vi "CSGaussmeter.saveSetting.vi"(0 "i ref in":refnum<vi>, 7 "ms timeout (10000)":i32=10000, 9 "setting path":string, 11 "error in (no error)":errorcluster) -> (4 "i ref out":refnum<vi>, 8 "timed out":bool, 15 "error out":errorcluster)   [LabVIEW 2014, in "CSGaussmeter.lvlib"]
uses:
  CSGaussmeter.lvlib
  CS_Core/CSObj/CSObj.lvlib
  CSlibraries/UtilityLib/UtilityLib.lvlib
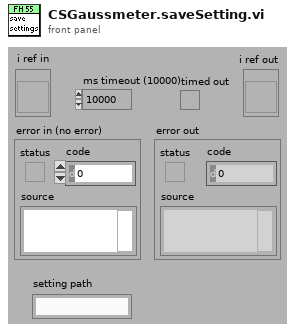
[diagram p1: front panel]
types:
  T1 = enum16{"open", "replace", "create", "open or create", "replace or create", "replace or create with confirmation"}
  T2 = typedef "CSGaussmeter.lvlib/CSGaussmeter.i attribute.ctl" = cluster{"Name":string, "VISA Resource Name":refnum<visa-resource-name>, "actValues":cluster{" Limit":bool, "Unit ":T3, "Temp_Unit":T4, "Max":T5, " Filter":bool, " Peak":bool, " Auto_Range":bool, "Range":T6, " Rel":bool, " CTemp":bool, " CField":bool, "AC_DC ":bool, "Set_lower":cluster{"Numeric":dbl, "Cancel Button":bool, "Unit":T7}, "Set_upper":cluster{"Numeric":dbl, "Cancel Button":bool, "Unit":T7}, "Set_Rel":cluster{"Numeric":dbl, "Cancel Button":bool, "Unit":T7}, "Zero":bool, " Local":bool, "Reset":bool, " Init":bool}, "FH 55 Gauss-/Teslameter":T8, "MAX_Value":T9, "MIN_Value":T9, "Rel_Value":T9, "Array ":string[], "LIMU":dbl, " LIML":dbl, "Messwerte 2":string, "Messwerte ":cluster{"Numeric":i32, "OK Button":bool}, "serviceID":cluster{"Current ID":i32, "Unit ID":i32, "Temp ID":i32, "Name ID \n":i32, "Visa ID ":i32}, "setValues ":cluster{" Limit":bool, "Unit ":T3, "Temp_Unit":T4, "Max":T5, " Filter":bool, " Peak":bool, " Auto_Range":bool, "Range":T6, " Rel":bool, " CTemp":bool, " CField":bool, "AC_DC ":bool, "Set_lower":cluster{"Numeric":dbl, "Cancel Button":bool, "Unit":T7}, "Set_upper":cluster{"Numeric":dbl, "Cancel Button":bool, "Unit":T7}, "Set_Rel":cluster{"Numeric":dbl, "Cancel Button":bool, "Unit":T7}, "Zero":bool, " Local":bool, "Reset":bool, " Init":bool}}
  T3 = typedef "FH 55.lvlib/Unit.ctl" = enum16{"T", "G", "A/m"}
  T4 = typedef "FH 55.lvlib/Temp_Unit.ctl" = enum16{"Temp off", "Celsius", "Fahrenheit"}
  T5 = typedef "FH 55.lvlib/Max.ctl" = enum16{"MAX off", "Show MAX", "MAX/MIN"}
  T6 = typedef "FH 55.lvlib/Range.ctl" = enum16{"1", "2", "3", "4", "5", "6", "7"}
  T7 = typedef "FH 55.lvlib/Unit2.ctl" = enum16{"mT", "G", "kA/m"}
  T8 = typedef "FH 55.lvlib/Display.ctl" = cluster{"current value":string, "Limit":string, "Remote":string, "function ":string, "Cluster":cluster{"AC/DC":string, "Auto":string, "Filter":string, "Range":string, "Rel":string, "Peak":string}}
  T9 = typedef "FH 55.lvlib/Value_String.ctl" = cluster{"Numeric":dbl, "String":string}
  T10 = cluster{" Limit":bool, "Unit ":T3, "Temp_Unit":T4, "Max":T5, " Filter":bool, " Peak":bool, " Auto_Range":bool, "Range":T6, " Rel":bool, " CTemp":bool, " CField":bool, "AC_DC ":bool, "Set_lower":cluster{"Numeric":dbl, "Cancel Button":bool, "Unit":T7}, "Set_upper":cluster{"Numeric":dbl, "Cancel Button":bool, "Unit":T7}, "Set_Rel":cluster{"Numeric":dbl, "Cancel Button":bool, "Unit":T7}, "Zero":bool, " Local":bool, "Reset":bool, " Init":bool}
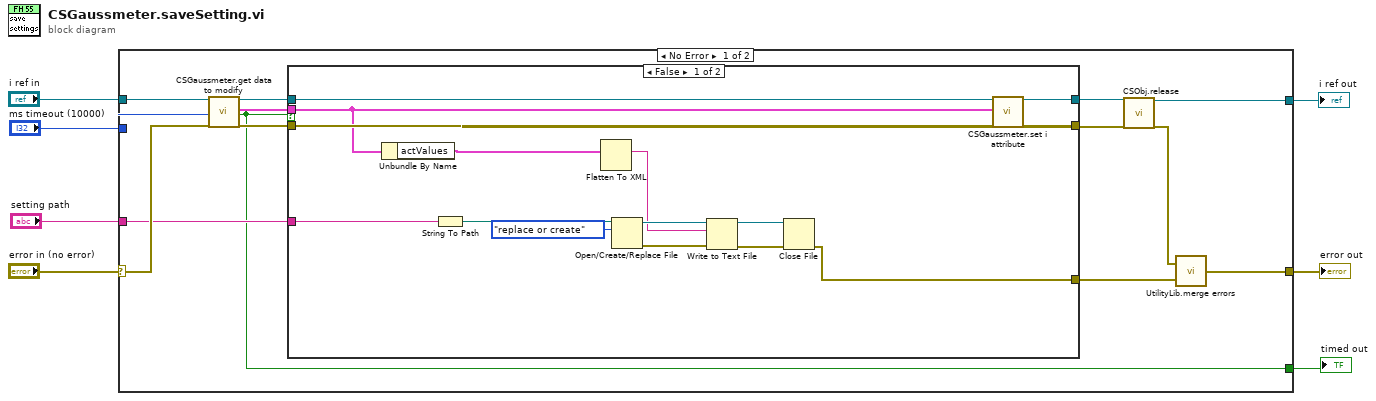
[diagram p0: block diagram]
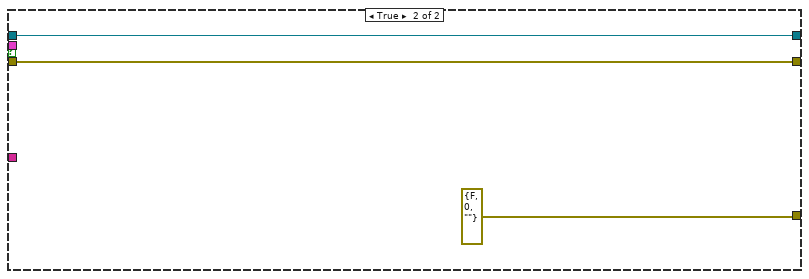
[diagram p2: hidden frame]
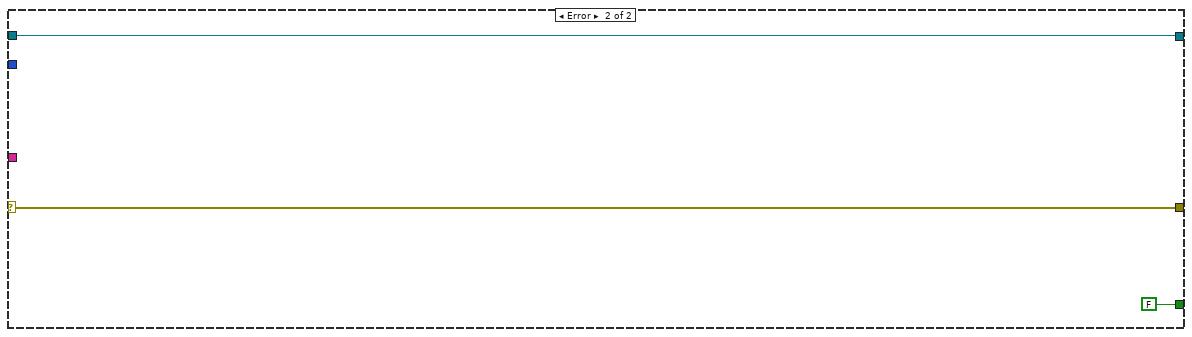
[diagram p3: hidden frame]
diagram:
  n1 = case shown="No Error" "error in (no error)" {
    selector: "error in (no error)" -> [w16 w41]
    tunnel: [w17 w41] -> w4
    tunnel: "i ref in" -> [w15 w42]
    tunnel: [w8 w42] -> w5
    tunnel: "ms timeout (10000)" -> [w10 _]
    tunnel: "setting path" -> [w11 _]
    tunnel: [w9 FALSE ("timed out")] -> w1
    frame No Error {
      n2 = call "CSGaussmeter.get data to modify.vi"("i ref in"=w15, "ms timeout (10000)"=w10, "error in (no error)"=w16) -> ("i ref out"=w14:refnum<vi>, "i attribute"=w13:T2, "timed out"=w9:bool, "error out"=w12:errorcluster)  [unwired: 13 in]
      n3 = case shown="False" w9 {
        tunnel: w14 -> [w36 w38]
        tunnel: w12 -> [w34 w39]
        tunnel: w13 -> [w32 _]
        tunnel: [w33 w39] -> w19
        tunnel: [w35 w38] -> w21
        tunnel: [w23 errorcluster {"status"=FALSE, "code"=0, "source"=""} ("error out")] -> w18
        tunnel: w11 -> [w22 _]
        frame False {
          n4 = Unbundle By Name(w32) -> ("actValues"=w31:T10)
          n5 = String To Path(string=w22) -> (path=w27:path)
          n6 = Flatten To XML(anything=w31) -> (xml string=w28:string)
          n7 = Open/Create/Replace File(file path (use dialog)=w27, operation (0:open)=T1."replace or create") -> (refnum out=w30:refnum<file>, error out=w29:errorcluster)  [unwired: 4 in, 1 out]
          n8 = Write to Text File(file (use dialog)=w30, text=w28, error in=w29) -> (refnum out=w25:refnum<file>, error out=w24:errorcluster)  [unwired: 1 in, 1 out]
          n9 = Close File(refnum=w25, error in=w24) -> (error out=w23:errorcluster)  [unwired: 1 out]
          n10 = call "CSGaussmeter.set i attribute.vi"("i ref in"=w36, "i attribute"=w32, "error in (no error)"=w34) -> ("i ref out"=w35:refnum<vi>, "error out"=w33:errorcluster)  [unwired: 15 in]
        }
        frame True {
        }
      }
      n11 = call "CSObj.release.vi"("i ref in"=w21, "error in (no error)"=w19) -> ("i ref out"=w8:refnum<vi>, "error out"=w20:errorcluster)  [unwired: 16 in]
      n12 = call "UtilityLib.merge errors.vi"("error2 (no error)"=w18, "error1 (no error)"=w20) -> ("error out"=w17:errorcluster)
    }
    frame Error {
    }
  }
  "i ref out" <- w5
  "error out" <- w4
  "timed out" <- w1
